vi "tcp_monitor_gen_frame.vi"(11 "DataString":string) -> (2 "length":i32, 3 "String":string)   [LabVIEW 2022 SP3]
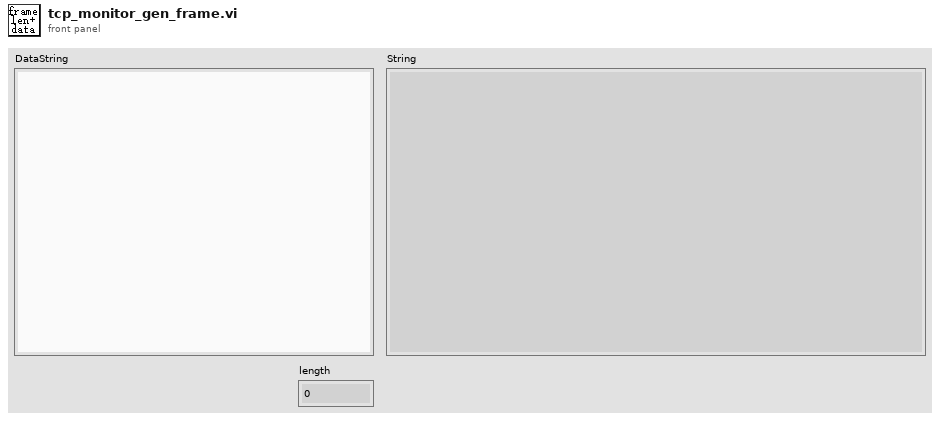
[diagram p1: front panel]
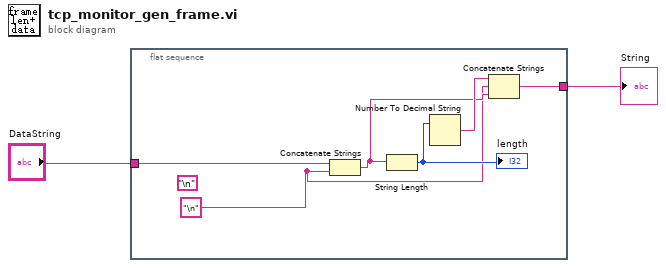
[diagram p0: block diagram]
diagram:
  n1 = flat-sequence {
    tunnel: "DataString" -> [w8]
    tunnel: [w4] -> w2
    frame #0 {
      (unwired) "\n"
      w3 = "\n"
      n2 = Concatenate Strings(w8, w3) -> (w5:string)
      n3 = String Length(string=w5) -> (length=w7:i32)
      "length" <- w7
      n4 = Number To Decimal String(number=w7) -> (decimal integer string=w6:string)  [unwired: 1 in]
      n5 = Concatenate Strings(w6, w3, w5) -> (w4:string)
    }
  }
  "String" <- w2
